vi "Scalar Inputs.vi"(8 "error in (no error)":errorcluster, 11 "Node Ptr":T1 format="%.0x") -> (0 "error out":errorcluster)   [LabVIEW 2019, in "FPGA Addon System Explorer.lvlib"]
uses:
  FPGA Addon System Explorer.lvlib
  <vilib>/NI VeriStand/Custom Device API/Custom Device Item Ref.ctl
  Types/SE UI Cluster.ctl
  Types/Channel Type.ctl
  Addon Shared/SubVIs/Constants.vi
  <vilib>/NI VeriStand/Custom Device API/Custom Device API.lvlib
  Addon Shared/FPGA Addon Shared.lvlib
panel:
  in  "remove":bool
  in  "add":bool
  in  "Available Registers":i32[](listbox)
  in  "Header 2":cluster{"Section Name":string}={"Section Name"="Register Settings"}
  in  "SHDocVw.IWebBrowser":refnum<k7>(container)
  in  "Header":cluster{"Section Name":string}={"Section Name"="Section Settings"}
  in  "Description":string
  out "Name":string
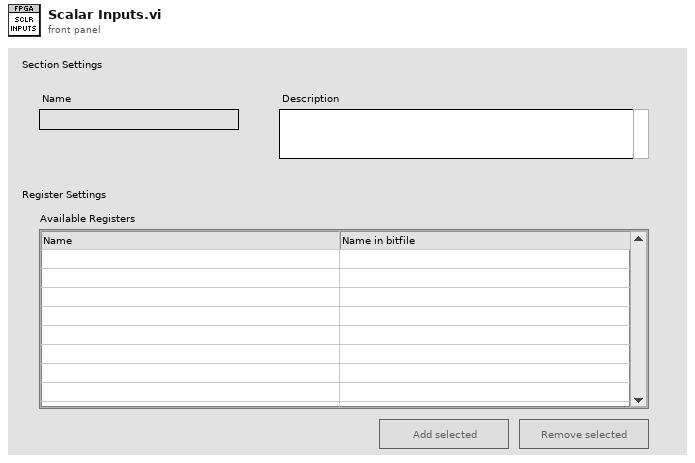
[diagram p1: front panel]
types:
  T1 = typedef "Custom Device API.lvlib/Custom Device Item Ref.ctl" = u64
  T2 = typedef "FPGA Addon System Explorer.lvlib/SE UI Cluster.ctl" = cluster{"Node Ptr":T1, "Add":refnum<vi>, "Remove":refnum<vi>, "Registers ListBox":refnum<vi>}
  T3 = typedef "Custom Device API.lvlib/Custom Device Item Info.ctl" = cluster{"Name":string, "Is Channel":bool, "GUID":string, "Is Waveform":bool}
  T4 = typedef "FPGA Addon System Explorer.lvlib/Channel Type.ctl" = enum16{"Write Channel", "Read Channel", "Write Waveform", "Read Waveform"}
  T5 = typedef "Custom Device API.lvlib/Custom Device Commands.ctl" = enum16{"Default", "Item renamed", "Shutdown", "Dynamic button pressed"}
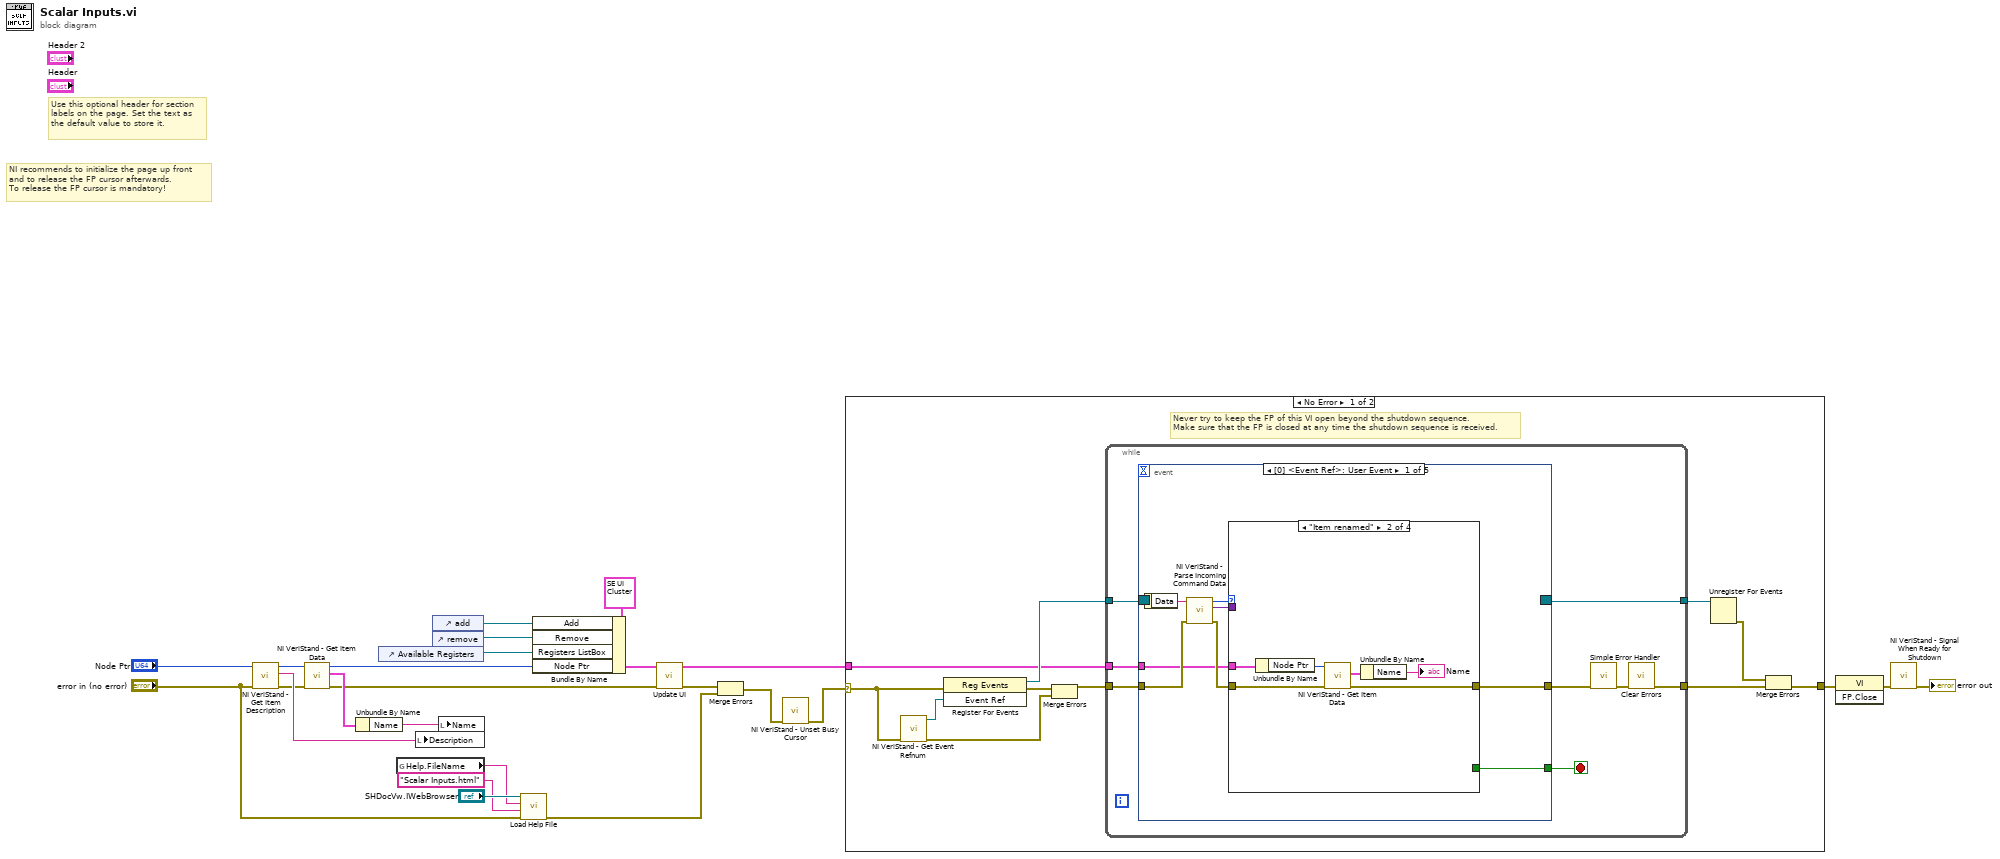
[diagram p0: block diagram]
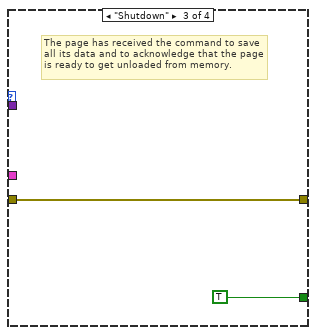
[diagram p3: hidden frame]
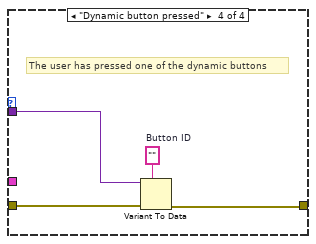
[diagram p4: hidden frame]
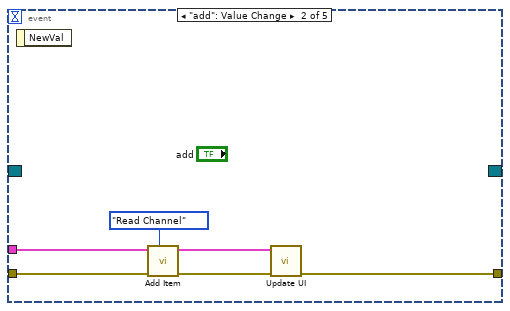
[diagram p5: hidden frame]
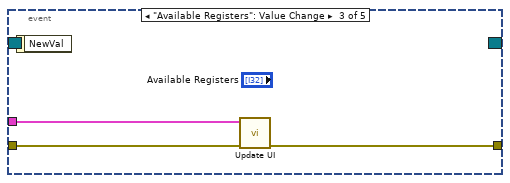
[diagram p6: hidden frame]
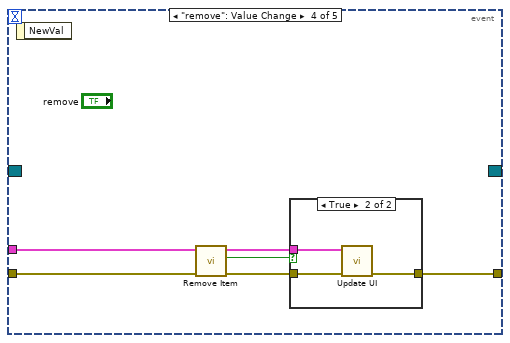
[diagram p7: hidden frame]
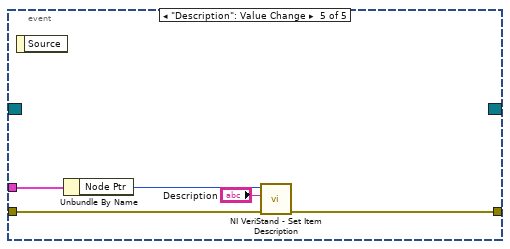
[diagram p9: hidden frame]
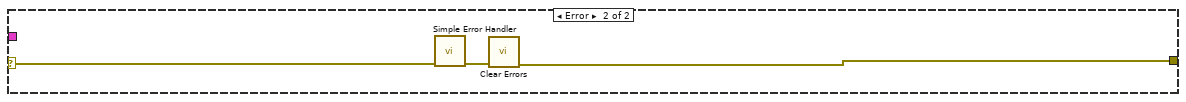
[diagram p10: hidden frame]
diagram:
  # "Use this optional header for section labels on the page. Set the text as the default value to store it."
  # "NI recommends to initialize the page up front\nand to release the FP cursor afterwards.\nTo release the FP cursor is mandatory!"
  n1 = call <vilib>:"NI VeriStand - Get Item Description.vi"("error in (no error)"="error in (no error)", "Item Ref in"="Node Ptr") -> ("error out"=w15:errorcluster, "Description"=w16:string, "Item Ref out"=w17:T1)  [unwired: 7 out]
  n2 = call <vilib>:"NI VeriStand - Get Item Data.vi"("error in (no error)"=w15, "Item Ref in"=w17) -> ("error out"=w12:errorcluster, "Item Info"=w14:T3, "Item Ref out"=w7:T1)  [unwired: 7 out]
  n3 = Unbundle By Name(w14) -> ("Name"=w13:string)
  n4 = control-ref of="Available Registers"() -> (w11:refnum<vi>)
  n5 = global read "Constants.vi" "Help.FileName"() -> (w19:string)
  n6 = local write "Description"(w16) -> ()
  n7 = control-ref of="add"() -> (w10:refnum<vi>)
  n8 = control-ref of="remove"() -> (w9:refnum<vi>)
  n9 = local write "Name"(w13) -> ()
  n10 = call "Load Help File.vi"("error in (no error)"="error in (no error)", "HTML File"="Scalar Inputs.html", "Main CHM File"=w19, "SHDocVw.IWebBrowser2"="SHDocVw.IWebBrowser") -> ("error out"=w4:errorcluster)  [unwired: 7 in]
  n11 = Bundle By Name(cluster=T2 {"Node Ptr"=18446744073709551615, "Add"=refnum, "Remove"=refnum, "Registers ListBox"=refnum} ("SE UI Cluster"), "Add"=w10, "Remove"=w9, "Registers ListBox"=w11, "Node Ptr"=w7) -> (w6:T2)
  n12 = call "Update UI.vi"("error in (no error)"=w12, "SE UI cluster in"=w6) -> ("error out"=w5:errorcluster, "SE UI cluster out"=w3:T2)  [unwired: 8 in]
  n13 = Merge Errors(w5, w4) -> (w2:errorcluster)
  n14 = call <vilib>:"NI VeriStand - Unset Busy Cursor.vi"("error in (no error)"=w2) -> ("error out"=w1:errorcluster)  [unwired: 10 out]
  n15 = case shown="No Error" w1 {
    selector: w1 -> [w33 w92]
    tunnel: [w26 w90] -> w25
    tunnel: w3 -> [w30 _]
    frame No Error {
      # "Never try to keep the FP of this VI open beyond the shutdown sequence.\nMake sure that the FP is closed at any time the shutdown sequence is received."
      n16 = call <vilib>:"NI VeriStand - Get Event Refnum.vi"("error in (no error)"=w33) -> ("error out"=w32:errorcluster, "Event Ref"=w34:refnum<user-event>)  [unwired: 9 out]
      n17 = register-events(error in=w33, w34) -> (reference out=w35:refnum<event-registration>, error out=w31:errorcluster)  [unwired: 1 in]
      n18 = Merge Errors(w31, w32) -> (w29:errorcluster)
      n19 = while {
        tunnel: w30 -> [w41]
        tunnel: w29 -> [w40]
        tunnel: w35 -> [w43]
        tunnel: [w44] -> w36
        tunnel: [w37] -> w28
        stop <- w42 stop-if-true
        n20 = event shown="[0] <Event Ref>: User Event" {
          selector: w43 -> [_ _ _ _ _]
          dyn-events: [_ _ _ _ _] -> w44
          timeout: _ -> [_ _ _ _ _]
          tunnel: [w49 _ _ _ _] -> w42
          tunnel: [w48 w67 w72 w77 w89] -> w38
          tunnel: w41 -> [w45 w70 w73 w79 w87]
          tunnel: w40 -> [w46 w69 w74 w80 w86]
          event User Event {
            n21 = event-data() -> ("Data"=w52:string)  [unwired: 1 out]
            n22 = call <vilib>:"NI VeriStand - Parse Incoming Command Data.vi"("error in (no error)"=w46, "Incoming data"=w52) -> ("error out"=w51:errorcluster, "Outgoing data"=w47:variant, "Action"=w50:T5)  [unwired: 7 out]
            n23 = case shown="\"Item renamed\"" w50 {
              tunnel: w51 -> [w53 w59 w60 w65]
              tunnel: [_ _ TRUE _] -> w49
              tunnel: [w53 w57 w60 w62] -> w48
              tunnel: w47 -> [_ _ _ w64]
              tunnel: w45 -> [_ w54 _ _]
              frame "Default", Default {
              }
              frame "Item renamed" {
                n24 = Unbundle By Name(w54) -> ("Node Ptr"=w56:T1)
                n25 = call <vilib>:"NI VeriStand - Get Item Data.vi"("error in (no error)"=w59, "Item Ref in"=w56) -> ("error out"=w57:errorcluster, "Item Info"=w58:T3)  [unwired: 8 out]
                n26 = Unbundle By Name(w58) -> ("Name"=→"Name":string)
              }
              frame "Shutdown" {
                # "The page has received the command to save all its data and to acknowledge that the page is ready to get unloaded from memory."
              }
              frame "Dynamic button pressed" {
                w63 = ""  # Button ID
                # "The user has pressed one of the dynamic buttons"
                n27 = Variant To Data(error in=w65, type=w63, Variant=w64) -> (error out=w62:errorcluster)  [unwired: 1 out]
              }
            }
          }
          event "add": Value Change {
            n28 = event-data() -> ()  [unwired: 2 out]
            n29 = call "Add Item.vi"("Action"=Channel_Type."Read Channel", "error in (no error)"=w69, "SE UI cluster in"=w70) -> ("error out"=w68:errorcluster, "SE UI cluster out"=w66:T2)  [unwired: 7 in]
            n30 = call "Update UI.vi"("error in (no error)"=w68, "SE UI cluster in"=w66) -> ("error out"=w67:errorcluster)  [unwired: 8 in, 1 out]
          }
          event "Available Registers": Value Change {
            n31 = event-data() -> ()  [unwired: 2 out]
            n32 = call "Update UI.vi"("error in (no error)"=w74, "SE UI cluster in"=w73) -> ("error out"=w72:errorcluster)  [unwired: 8 in, 1 out]
          }
          event "remove": Value Change {
            n33 = event-data() -> ()  [unwired: 2 out]
            n34 = call "Remove Item.vi"("error in (no error)"=w80, "SE UI cluster in"=w79) -> ("error out"=w78:errorcluster, "Deleted?"=w75:bool, "SE UI cluster out"=w76:T2)  [unwired: 7 in]
            n35 = case shown="True" w75 {
              tunnel: w78 -> [w81 w84]
              tunnel: [w81 w83] -> w77
              tunnel: w76 -> [_ w82]
              frame False {
              }
              frame True {
                n36 = call "Update UI.vi"("error in (no error)"=w84, "SE UI cluster in"=w82) -> ("error out"=w83:errorcluster)  [unwired: 8 in, 1 out]
              }
            }
          }
          event "Description": Value Change {
            n37 = event-data() -> ()  [unwired: 2 out]
            n38 = Unbundle By Name(w87) -> ("Node Ptr"=w85:T1)
            n39 = call <vilib>:"NI VeriStand - Set Item Description.vi"("error in (no error)"=w86, "Description"="Description", "Item Ref in"=w85) -> ("error out"=w89:errorcluster)  [unwired: 8 out]
          }
        }
        n40 = call <vilib>:"Simple Error Handler.vi"("error in (no error)"=w38) -> ("error out"=w39:errorcluster)  [unwired: 1 in, 7 out]
        n41 = call <vilib>:"Clear Errors.vi"("error in (no error)"=w39) -> ("error out"=w37:errorcluster)  [unwired: 1 in, 5 out]
      }
      n42 = Unregister For Events(event registration refnum=w36) -> (error out=w27:errorcluster)  [unwired: 1 in]
      n43 = Merge Errors(w27, w28) -> (w26:errorcluster)
    }
    frame Error {
      n44 = call <vilib>:"Simple Error Handler.vi"("error in (no error)"=w92) -> ("error out"=w91:errorcluster)  [unwired: 1 in, 7 out]
      n45 = call <vilib>:"Clear Errors.vi"("error in (no error)"=w91) -> ("error out"=w90:errorcluster)  [unwired: 1 in, 5 out]
    }
  }
  n46 = invoke class="VI" method="FP.Close"(error in=w25) -> (error out=w24:errorcluster)  [unwired: 2 in, 2 out]
  n47 = call <vilib>:"NI VeriStand - Signal When Ready for Shutdown.vi"("error in (no error)"=w24) -> ("error out"=→"error out":errorcluster)  [unwired: 10 out]
